vi "RobotTurnMovement.vi"(9 "index":i32=5, 10 "Current Image Array":i32[](array[numeric])=[0, 0, 0, 0, 0, 0, 0, 0, 0, 0, 0, 0, 0, 0, 0, 0, 0, 0], 11 "VISA Refnum in":refnum<visa-resource-name>="COM6") -> (0 "error out":errorcluster, 1 "Image Value":i32, 2 "Output Array":i32[](array[numeric]), 3 "VISA Refnum out":refnum<visa-resource-name>)   [LabVIEW 2018]
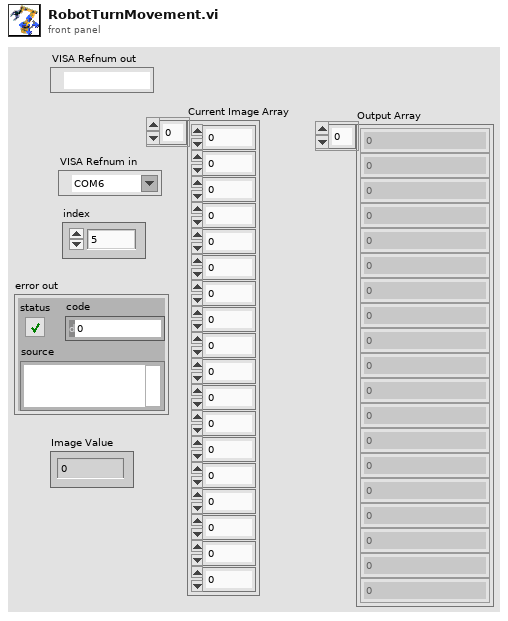
[diagram p1: front panel]
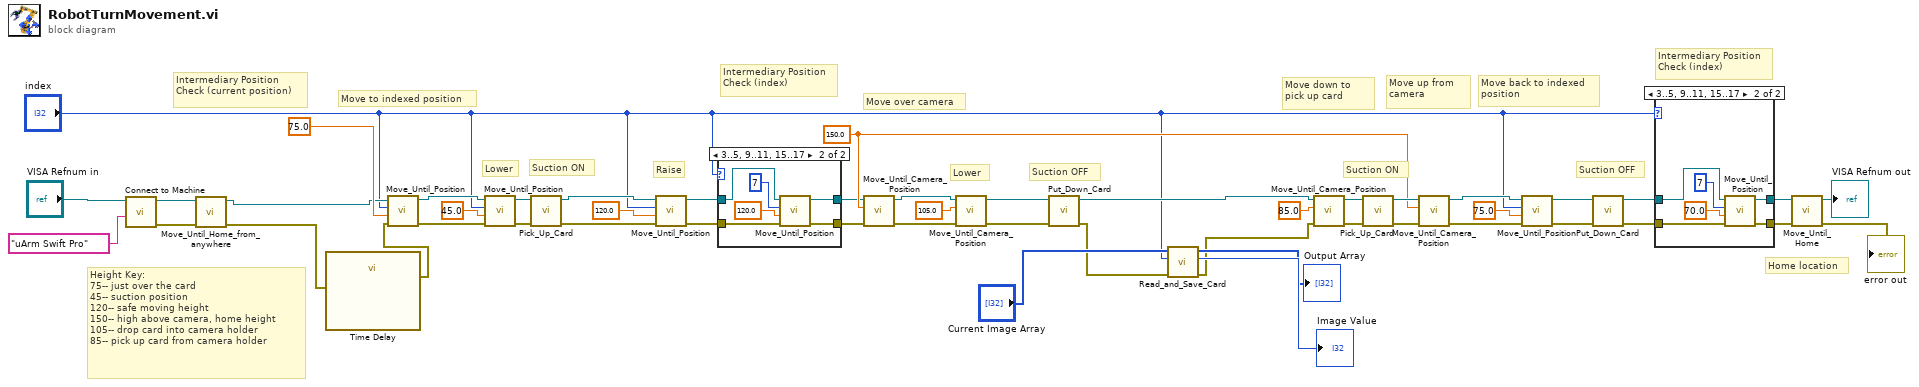
[diagram p0: block diagram]
diagram:
  w37 = 150.0 ("Desired Height")
  # "Height Key:\n75-- just over the card\n45-- suction position\n120-- safe moving height\n150-- high above camera, home height\n105-- drop card into camera holder\n85-- pick up card from camera holder"
  # "Intermediary Position\nCheck (index)"
  # "Suction ON"
  # "Intermediary Position Check (index)"
  # "Intermediary Position Check (current position)"
  # "Raise"
  # "Lower"
  # "Move back to indexed position"
  # "Lower"
  # "Move to indexed position"
  # "Home location"
  # "Suction ON"
  # "Move down to pick up card"
  # "Suction OFF"
  # "Suction OFF"
  # "Move up from camera"
  # "Move over camera"
  n1 = call "Connect to Machine .vi"("Firmware"="uArm Swift Pro", "Machine In"="VISA Refnum in") -> ("error out"=w11:errorcluster, "Machine Out"=w12:refnum<visa-resource-name>)  [unwired: 7 in, 1 out]
  n2 = call "Move_Until_Home_from_anywhere.vi"("error in"=w11, "Machine In"=w12) -> ("error out"=w9:errorcluster, "Machine Out"=w10:refnum<visa-resource-name>)  [unwired: 8 in]
  n3 = call "Time Delay"("error in (no error)"=w9) -> ("error out"=w8:errorcluster)  [unwired: 10 in]
  n4 = call "Move_Until_Position.vi"("error in (no error)"=w8, "Z-Position"=75.0, "index"="index", "VISA Refnum in"=w10) -> ("error out"=w35:errorcluster, "VISA Refnum out"=w36:refnum<visa-resource-name>)  [unwired: 6 in]
  n5 = call "Move_Until_Position.vi"("error in (no error)"=w35, "Z-Position"=45.0, "index"="index", "VISA Refnum in"=w36) -> ("error out"=w19:errorcluster, "VISA Refnum out"=w20:refnum<visa-resource-name>)  [unwired: 6 in]
  n6 = call "Pick_Up_Card.vi"("error in"=w19, "VISA Refnum in"=w20) -> ("error out"=w17:errorcluster, "Machine Out"=w18:refnum<visa-resource-name>)  [unwired: 6 in]
  n7 = call "Move_Until_Position.vi"("error in (no error)"=w17, "Z-Position"=120.0, "index"="index", "VISA Refnum in"=w18) -> ("error out"=w25:errorcluster, "VISA Refnum out"=w26:refnum<visa-resource-name>)  [unwired: 6 in]
  n8 = case shown="3..5, 9..11, 15..17" "index" {
    tunnel: [w51 w55] -> w24
    tunnel: [w50 w54] -> w23
    tunnel: w26 -> [w51 w53]
    tunnel: w25 -> [w50 w52]
    frame 0, Default {
    }
    frame 3..5, 9..11, 15..17 {
      n9 = call "Move_Until_Position.vi"("error in (no error)"=w52, "Z-Position"=120.0, "index"=7, "VISA Refnum in"=w53) -> ("error out"=w54:errorcluster, "VISA Refnum out"=w55:refnum<visa-resource-name>)  [unwired: 6 in]
    }
  }
  n10 = call "Move_Until_Camera_Position.vi"("error in (no error)"=w23, "Desired Height"=w37, "VISA Refnum in"=w24) -> ("error out"=w32:errorcluster, "VISA Refnum out"=w31:refnum<visa-resource-name>)  [unwired: 7 in]
  n11 = call "Move_Until_Camera_Position.vi"("error in (no error)"=w32, "Desired Height"=105.0, "VISA Refnum in"=w31) -> ("error out"=w16:errorcluster, "VISA Refnum out"=w30:refnum<visa-resource-name>)  [unwired: 7 in]
  n12 = call "Put_Down_Card.vi"("error in"=w16, "VISA Refnum in"=w30) -> ("error out"=w3:errorcluster, "Machine Out"=w44:refnum<visa-resource-name>)  [unwired: 7 in]
  n13 = call "Read_and_Save_Card.vi"("error in (no error)"=w3, "index"="index", "Current Image Array"="Current Image Array") -> ("error out"=w2:errorcluster, "Image Value"=→"Image Value":i32, "Output Image Array"=→"Output Array":i32[])  [unwired: 6 in]
  n14 = call "Move_Until_Camera_Position.vi"("error in (no error)"=w2, "Desired Height"=85.0, "VISA Refnum in"=w44) -> ("error out"=w45:errorcluster, "VISA Refnum out"=w46:refnum<visa-resource-name>)  [unwired: 7 in]
  n15 = call "Pick_Up_Card.vi"("error in"=w45, "VISA Refnum in"=w46) -> ("error out"=w40:errorcluster, "Machine Out"=w41:refnum<visa-resource-name>)  [unwired: 6 in]
  n16 = call "Move_Until_Camera_Position.vi"("error in (no error)"=w40, "Desired Height"=w37, "VISA Refnum in"=w41) -> ("error out"=w39:errorcluster, "VISA Refnum out"=w38:refnum<visa-resource-name>)  [unwired: 7 in]
  n17 = call "Move_Until_Position.vi"("error in (no error)"=w39, "Z-Position"=75.0, "index"="index", "VISA Refnum in"=w38) -> ("error out"=w15:errorcluster, "VISA Refnum out"=w42:refnum<visa-resource-name>)  [unwired: 6 in]
  n18 = call "Put_Down_Card.vi"("error in"=w15, "VISA Refnum in"=w42) -> ("error out"=w14:errorcluster, "Machine Out"=w22:refnum<visa-resource-name>)  [unwired: 7 in]
  n19 = case shown="3..5, 9..11, 15..17" "index" {
    tunnel: [w59 w63] -> w21
    tunnel: w22 -> [w59 w62]
    tunnel: w14 -> [w58 w61]
    tunnel: [w58 w60] -> w13
    frame 0, Default {
    }
    frame 3..5, 9..11, 15..17 {
      n20 = call "Move_Until_Position.vi"("error in (no error)"=w61, "Z-Position"=70.0, "index"=7, "VISA Refnum in"=w62) -> ("error out"=w60:errorcluster, "VISA Refnum out"=w63:refnum<visa-resource-name>)  [unwired: 6 in]
    }
  }
  n21 = call "Move_Until_Home.vi"("error in (no error)"=w13, "VISA Refnum in"=w21) -> ("error out"=→"error out":errorcluster, "VISA Refnum out"=→"VISA Refnum out":refnum<visa-resource-name>)  [unwired: 8 in]
